vi "ANDOR_GetEMGainRange.vi"(8 "error in (no error)":errorcluster) -> (0 "error out":errorcluster, 1 "DLL error code":u32, 2 "high":i32, 3 "low":i32, 5 "EM Gain Range":cluster{"low":i32, "high":i32})   [LabVIEW 2010]
doc: "Returns the minimum and maximum values of the current selected EM Gain mode and temperature of the sensor.\n\n<B>Parameters:</B>\nint* low: lowest gain setting\nint* high: highest gain setting.\n\n<B>Error codes:</B>\nDRV_SUCCESS Detector size returned.\nDRV_NOT_INITIALIZED System not initialized.\nDRV_ACQUIRING Acquisition in progress."
uses:
  Program Files/Andor SOLIS/atmcd32d.dll
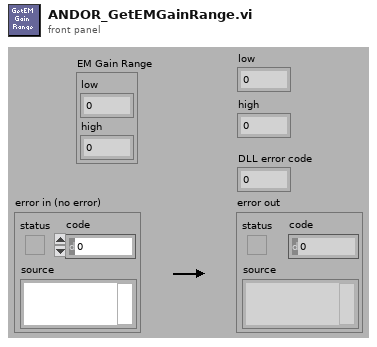
[diagram p1: front panel]
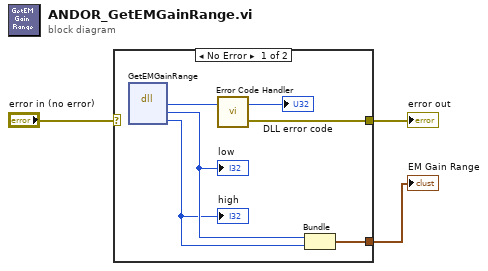
[diagram p0: block diagram]
diagram:
  n1 = case shown="No Error" "error in (no error)" {
    selector: "error in (no error)" -> [_ w10]
    tunnel: [w8 w10] -> w2
    tunnel: [w4 _] -> w1
    frame No Error {
      n2 = dll-call lib="C:/Program Files/Andor SOLIS/atmcd32d.dll" fn="GetEMGainRange"() -> ("return type"=w9:u32, "xpixels"=w6:i32, "ypixels"=w5:i32)  [unwired: 5 in, 2 out]
      "low" <- w6
      "high" <- w5
      n3 = call <userlib>:"Error Code Handler.vi"("DLL error code"=w9) -> ("error out"=w8:errorcluster, "dup DLL error code"=→"DLL error code":u32)  [unwired: 1 in]
      n4 = Bundle("xpixels"=w6, "ypixels"=w5) -> (w4:cluster{"xpixels":i32, "ypixels":i32})  [unwired: 1 in]
    }
    frame Error {
    }
  }
  "error out" <- w2
  "EM Gain Range" <- w1
